vi "Add Control Refnum From Control.vi"(6 "Variant in":variant, 7 "Shift Pressed?":bool, 8 "error in (no error)":errorcluster, 10 "QD Combo Box Ref":refnum<vi>, 11 "QD Launch VI Ref":refnum<vi>) -> (0 "error out":errorcluster, 4 "Variant out":variant)   [LabVIEW 2015]
doc: "PLUGIN_DESCRIPTION: Clones the selected Control(s) or Indicator(s) on the Front Panel but changes Controls to Indicators and vice versa. In addition, if found on the Connector Pane, will attempt to place the newly created control on the opposite (left / right) side of the Connector Pane.\nNote: This script only supports the following patterns: 4x2x2x4, 5x3x3x5, 6x4x4x6, and 8x6x6x8.\n\nIf you rotate your connector panes - this script is not for you!\n\nPLUGIN_DEFAULT_SHORTCUT: C"
uses:
  <vilib>/Utility/traverseref.llb/TRef TravTarget.ctl
  <vilib>/Utility/traverseref.llb/VI Scripting - Traverse.lvlib
panel:
  in  "Undo Name":string="Dup Con I/O"
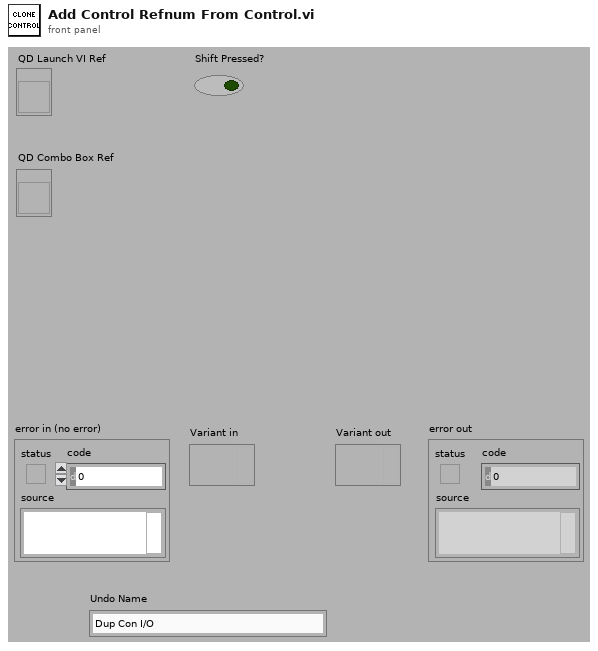
[diagram p1: front panel]
types:
  T1 = typedef "TRef TravTarget.ctl" = enum16{"FP", "BD", "Other"}
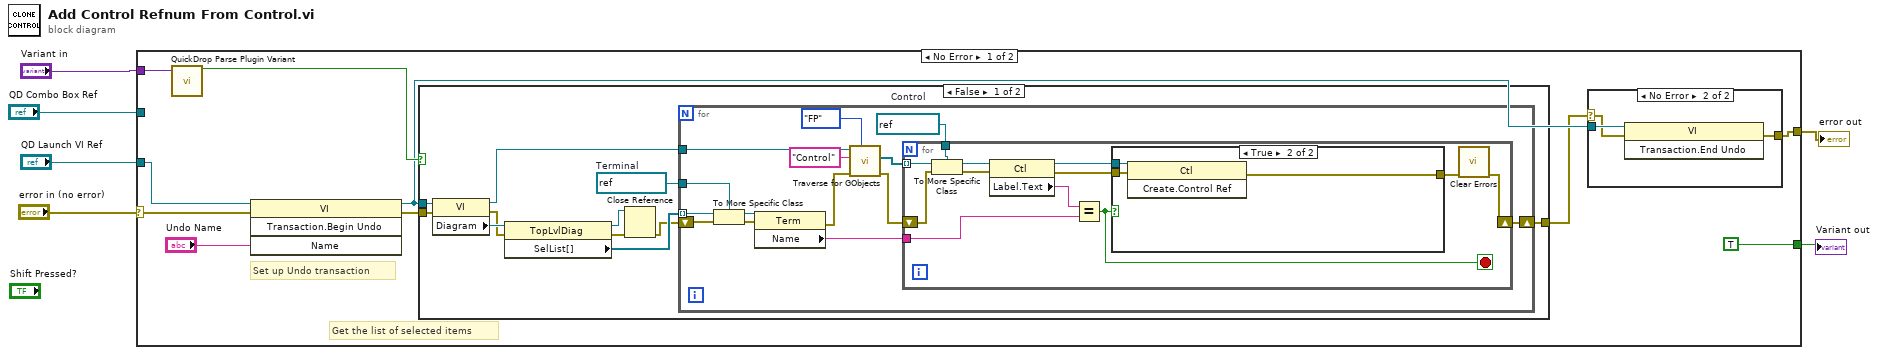
[diagram p0: block diagram]
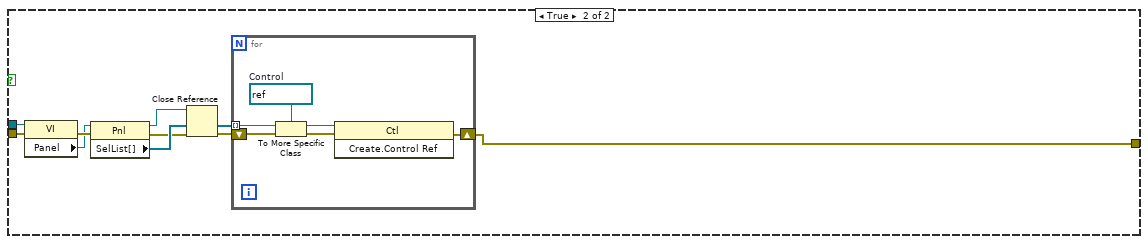
[diagram p3: hidden frame]
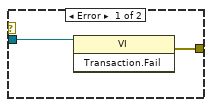
[diagram p4: hidden frame]
diagram:
  n1 = case shown="No Error" "error in (no error)" {
    selector: "error in (no error)" -> [w15 w78]
    tunnel: [w12 w78] -> w3
    tunnel: "QD Combo Box Ref" -> [_ _]
    tunnel: "QD Launch VI Ref" -> [w14 _]
    tunnel: "Variant in" -> [w11 _]
    tunnel: [TRUE _] -> w1
    frame No Error {
      # "Get the list of selected items"
      # "Set up Undo transaction"
      n2 = call <vilib>:"QuickDrop Parse Plugin Variant.vi"("QDKS Variant in"=w11) -> ("QD Launch VI Panel?"=w10:bool)  [unwired: 12 in, 2 out]
      n3 = invoke class="VI" method="Transaction.Begin Undo"(reference=w14, error in=w15, "Name"="Undo Name") -> (reference out=w9:refnum<vi>, error out=w13:errorcluster)  [unwired: 1 in, 2 out]
      n4 = case shown="False" w10 {
        tunnel: w13 -> [w26 w64]
        tunnel: w9 -> [w27 w63]
        tunnel: [w22 w61] -> w7
        frame False {
          w17 = refnum<vi> refnum  # Terminal
          n5 = property class="VI"(reference=w27, error in=w26) -> (reference out=w18:refnum<vi>, error out=w24:errorcluster, "Diagram"=w25:refnum<vi>)
          n6 = property class="TopLvlDiag"(reference=w25, error in=w24) -> (reference out=w19:refnum<vi>, error out=w21:errorcluster, "SelList[]"=w23:refnum<vi>[])
          n7 = Close Reference(reference=w19, error in (no error)=w21) -> (error out=w20:errorcluster)
          n8 = for {
            tunnel: w23 -> [w41] mode=indexing
            shift-right: [w29] -> w22
            shift-left: w20 -> [w40]
            tunnel: w18 -> [w36]
            tunnel: w17 -> [w37]
            w32 = refnum<vi> refnum  # Control
            n9 = To More Specific Class(target class=w37, reference=w41, error in=w40) -> (specific class reference=w39:refnum<vi>, error out=w38:errorcluster)
            n10 = property class="Term"(reference=w39, error in=w38) -> (error out=w34:errorcluster, "Name"=w30:string)  [unwired: 1 out]
            n11 = call <vilib>:"Traverse for GObjects.vi"("Traverse Target"=TRef_TravTarget."FP", "error in (no error)"=w34, "Class Name"="Control", "VI Refnum"=w36) -> ("error out"=w31:errorcluster, "References"=w33:refnum<vi>[])  [unwired: 4 in, 2 out]
            n12 = for {
              tunnel: w33 -> [w53] mode=indexing
              tunnel: w32 -> [w52]
              tunnel: w30 -> [w47]
              shift-right: [w43] -> w29
              shift-left: w31 -> [w51]
              stop <- w42 stop-if-true
              n13 = To More Specific Class(target class=w52, reference=w53, error in=w51) -> (specific class reference=w50:refnum<vi>, error out=w49:errorcluster)
              n14 = property class="Ctl"(reference=w50, error in=w49) -> (reference out=w46:refnum<vi>, error out=w45:errorcluster, "Label.Text"=w48:string)
              n15 = Equal?(x=w48, y=w47) -> (x = y?=w42:bool)
              n16 = case shown="True" w42 {
                tunnel: w46 -> [_ w57]
                tunnel: w45 -> [w54 w56]
                tunnel: [w54 w55] -> w44
                frame False {
                }
                frame True {
                  n17 = invoke class="Ctl" method="Create.Control Ref"(reference=w57, error in=w56) -> (error out=w55:errorcluster)  [unwired: 1 in, 2 out]
                }
              }
              n18 = call <vilib>:"Clear Errors.vi"("error in (no error)"=w44) -> ("error out"=w43:errorcluster)  [unwired: 5 in, 1 out]
            }
          }
        }
        frame True {
          n19 = property class="VI"(reference=w63, error in=w64) -> (error out=w66:errorcluster, "Panel"=w65:refnum<vi>)  [unwired: 1 out]
          n20 = property class="Pnl"(reference=w65, error in=w66) -> (reference out=w58:refnum<vi>, error out=w60:errorcluster, "SelList[]"=w62:refnum<vi>[])
          n21 = Close Reference(reference=w58, error in (no error)=w60) -> (error out=w59:errorcluster)
          n22 = for {
            tunnel: w62 -> [w72] mode=indexing
            shift-right: [w67] -> w61
            shift-left: w59 -> [w70]
            w71 = refnum<vi> refnum  # Control
            n23 = To More Specific Class(target class=w71, reference=w72, error in=w70) -> (specific class reference=w69:refnum<vi>, error out=w68:errorcluster)
            n24 = invoke class="Ctl" method="Create.Control Ref"(reference=w69, error in=w68) -> (error out=w67:errorcluster)  [unwired: 1 in, 2 out]
          }
        }
      }
      n25 = case shown="No Error" w7 {
        selector: w7 -> [_ w75]
        tunnel: [w74 w77] -> w12
        tunnel: w9 -> [w73 w76]
        frame Error {
          n26 = invoke class="VI" method="Transaction.Fail"(reference=w73) -> (error out=w74:errorcluster)  [unwired: 2 in, 2 out]
        }
        frame No Error {
          n27 = invoke class="VI" method="Transaction.End Undo"(reference=w76, error in=w75) -> (error out=w77:errorcluster)  [unwired: 1 in, 2 out]
        }
      }
    }
    frame Error {
    }
  }
  "error out" <- w3
  "Variant out" <- w1
